vi "Read MasterConfiguration.vi"(7 "Action (Rd)":enum16{"Read", "Write"}(ring)=enum."Write", 8 "error in (no error)":errorcluster, 10 "MasterConfiguration":T1={"E109Configuration"={"PodPorts"=[{"portID"=101, "LocationID"="PodIn", "locationIndex"=1}, {"portID"=102, "LocationID"="PodOut", "locationIndex"=2}], "PodLocations"=["Buffer1", "Buffer2", "Buffer3", "Buffer4", "Buffer5", "Buffer6", "Buffer7", "Buffer8", "Buffer9", "Buffer10", "Buffer11", "Buffer12", "Buffer13", "Buffer14", "Buffer15", "Buffer16", "ASML1", "ASML2", "Manual"], "ReticleLocations"=[], "Opener1LocationID"="", "Opener2LocationID"="", "PodGantryArmLocationID"="", "VariableListPath"="", "EPJFilepath"=""}, "InBound"={"Simulation"=FALSE, "E84 Port Setup"={"Port ID"="", "baud rate"=9600, "data bits"=8, "parity"=enum."None", "stop bits"=10, "flow control"=0}, "UseVISAEvents"=FALSE, "Name"=""}, "OutBound"={"Simulation"=FALSE, "E84 Port Setup"={"Port ID"="", "baud rate"=9600, "data bits"=8, "parity"=enum."None", "stop bits"=10, "flow control"=0}, "UseVISAEvents"=FALSE, "Name"=""}, "InboundPodID"={"Simulation"=FALSE, "LoadPortCOM"={"VISA"="", "baud rate"=0, "data bits"=0, "parity"=enum."None", "flow control"=enum."None"}, "RFIDCOM"={"VISA"="", "baud rate"=0, "data bits"=0, "parity"=enum."None", "flow control"=enum."None"}, "SimulationRFID"=FALSE}, "OutboundPodID"={"Simulation"=FALSE, "LoadPortCOM"={"VISA"="", "baud rate"=0, "data bits"=0, "parity"=enum."None", "flow control"=enum."None"}, "RFIDCOM"={"VISA"="", "baud rate"=0, "data bits"=0, "parity"=enum."None", "flow control"=enum."None"}, "SimulationRFID"=FALSE}, "PBInterface"={"Simulation"=FALSE, "IPAddress"="", "StatusTag"="", "APIMoveTag"=""}} {"OutBound"."E84 Port Setup"."baud rate" items=["75"=75, "110"=110, "134"=134, "150"=150, "300"=300, "600"=600, "1200"=1200, "1800"=1800, "2400"=2400, "4800"=4800, "7200"=7200, "9600"=9600, "14400"=14400, "19200"=19200, "28800"=28800, "38400"=38400, "56000"=56000, "57600"=57600, "115200"=115200, "128000"=128000, "230400"=230400]; "OutBound"."E84 Port Setup"."flow control" items=["None", "XON/XOFF", "RTS/CTS", "XON/XOFF & RTS/CTS", "DTR/DSR", "XON/XOFF & DTR/DSR"]; "OutBound"."E84 Port Setup"."stop bits" items=["1"=10, "1.5"=15, "2"=20]; "OutBound"."E84 Port Setup"."data bits" min=5 max=8 step=1; "InBound"."E84 Port Setup"."baud rate" items=["75"=75, "110"=110, "134"=134, "150"=150, "300"=300, "600"=600, "1200"=1200, "1800"=1800, "2400"=2400, "4800"=4800, "7200"=7200, "9600"=9600, "14400"=14400, "19200"=19200, "28800"=28800, "38400"=38400, "56000"=56000, "57600"=57600, "115200"=115200, "128000"=128000, "230400"=230400]; "InBound"."E84 Port Setup"."flow control" items=["None", "XON/XOFF", "RTS/CTS", "XON/XOFF & RTS/CTS", "DTR/DSR", "XON/XOFF & DTR/DSR"]; "InBound"."E84 Port Setup"."stop bits" items=["1"=10, "1.5"=15, "2"=20]; "InBound"."E84 Port Setup"."data bits" min=5 max=8 step=1}, 11 "ConfigFile":path) -> (0 "error out":errorcluster, 2 "MasterConfigOut":T1={"E109Configuration"={"PodPorts"=[{"portID"=101, "LocationID"="PodIn", "locationIndex"=1}, {"portID"=102, "LocationID"="PodOut", "locationIndex"=2}], "PodLocations"=["Buffer1", "Buffer2", "Buffer3", "Buffer4", "Buffer5", "Buffer6", "Buffer7", "Buffer8", "Buffer9", "Buffer10", "Buffer11", "Buffer12", "Buffer13", "Buffer14", "Buffer15", "Buffer16", "ASML1", "ASML2", "Manual"], "ReticleLocations"=[], "Opener1LocationID"="", "Opener2LocationID"="", "PodGantryArmLocationID"="", "VariableListPath"="", "EPJFilepath"=""}, "InBound"={"Simulation"=FALSE, "E84 Port Setup"={"Port ID"="", "baud rate"=9600, "data bits"=8, "parity"=enum."None", "stop bits"=10, "flow control"=0}, "UseVISAEvents"=FALSE, "Name"=""}, "OutBound"={"Simulation"=FALSE, "E84 Port Setup"={"Port ID"="", "baud rate"=9600, "data bits"=8, "parity"=enum."None", "stop bits"=10, "flow control"=0}, "UseVISAEvents"=FALSE, "Name"=""}, "InboundPodID"={"Simulation"=FALSE, "LoadPortCOM"={"VISA"="", "baud rate"=0, "data bits"=0, "parity"=enum."None", "flow control"=enum."None"}, "RFIDCOM"={"VISA"="", "baud rate"=0, "data bits"=0, "parity"=enum."None", "flow control"=enum."None"}, "SimulationRFID"=FALSE}, "OutboundPodID"={"Simulation"=FALSE, "LoadPortCOM"={"VISA"="", "baud rate"=0, "data bits"=0, "parity"=enum."None", "flow control"=enum."None"}, "RFIDCOM"={"VISA"="", "baud rate"=0, "data bits"=0, "parity"=enum."None", "flow control"=enum."None"}, "SimulationRFID"=FALSE}, "PBInterface"={"Simulation"=FALSE, "IPAddress"="", "StatusTag"="", "APIMoveTag"=""}} {"OutBound"."E84 Port Setup"."baud rate" items=["75"=75, "110"=110, "134"=134, "150"=150, "300"=300, "600"=600, "1200"=1200, "1800"=1800, "2400"=2400, "4800"=4800, "7200"=7200, "9600"=9600, "14400"=14400, "19200"=19200, "28800"=28800, "38400"=38400, "56000"=56000, "57600"=57600, "115200"=115200, "128000"=128000, "230400"=230400]; "OutBound"."E84 Port Setup"."flow control" items=["None", "XON/XOFF", "RTS/CTS", "XON/XOFF & RTS/CTS", "DTR/DSR", "XON/XOFF & DTR/DSR"]; "OutBound"."E84 Port Setup"."stop bits" items=["1"=10, "1.5"=15, "2"=20]; "OutBound"."E84 Port Setup"."data bits" min=5 max=8 step=1; "InBound"."E84 Port Setup"."baud rate" items=["75"=75, "110"=110, "134"=134, "150"=150, "300"=300, "600"=600, "1200"=1200, "1800"=1800, "2400"=2400, "4800"=4800, "7200"=7200, "9600"=9600, "14400"=14400, "19200"=19200, "28800"=28800, "38400"=38400, "56000"=56000, "57600"=57600, "115200"=115200, "128000"=128000, "230400"=230400]; "InBound"."E84 Port Setup"."flow control" items=["None", "XON/XOFF", "RTS/CTS", "XON/XOFF & RTS/CTS", "DTR/DSR", "XON/XOFF & DTR/DSR"]; "InBound"."E84 Port Setup"."stop bits" items=["1"=10, "1.5"=15, "2"=20]; "InBound"."E84 Port Setup"."data bits" min=5 max=8 step=1})   [LabVIEW 2020]
uses:
  Controls/TD MasterConfiguration--cluster.ctl
  Subsystems/Cimetrix-main/Classes/TopLevel/Typedefs/E109Configuration--Cluster.ctl
  Subsystems/Cimetrix-main/Classes/TopLevel/Typedefs/E109_API_CreatePodPort_Data--Cluster.ctl
  Subsystems/Cimetrix-main/Classes/TopLevel/Typedefs/ToolModuleConfig--Cluster.ctl
  Subsystems/E84LoadPort/DataTypes/Settings--cluster.ctl
  Seminet_Common/DataTypes/serial_port_setup.ctl
  Subsystems/LoadPort/DataTypes/Settings--cluster.ctl
  Controls/TD SerialPortConfig--Cluster.ctl
  Subsystems/PodBufferInterface/DataTypes/Settings--cluster.ctl
  Subsystems/E84LoadPort/E84LoadPort.lvclass
  Subsystems/LoadPort/LoadPort.lvclass
  Subsystems/PodBufferInterface/PodBufferInterface.lvclass
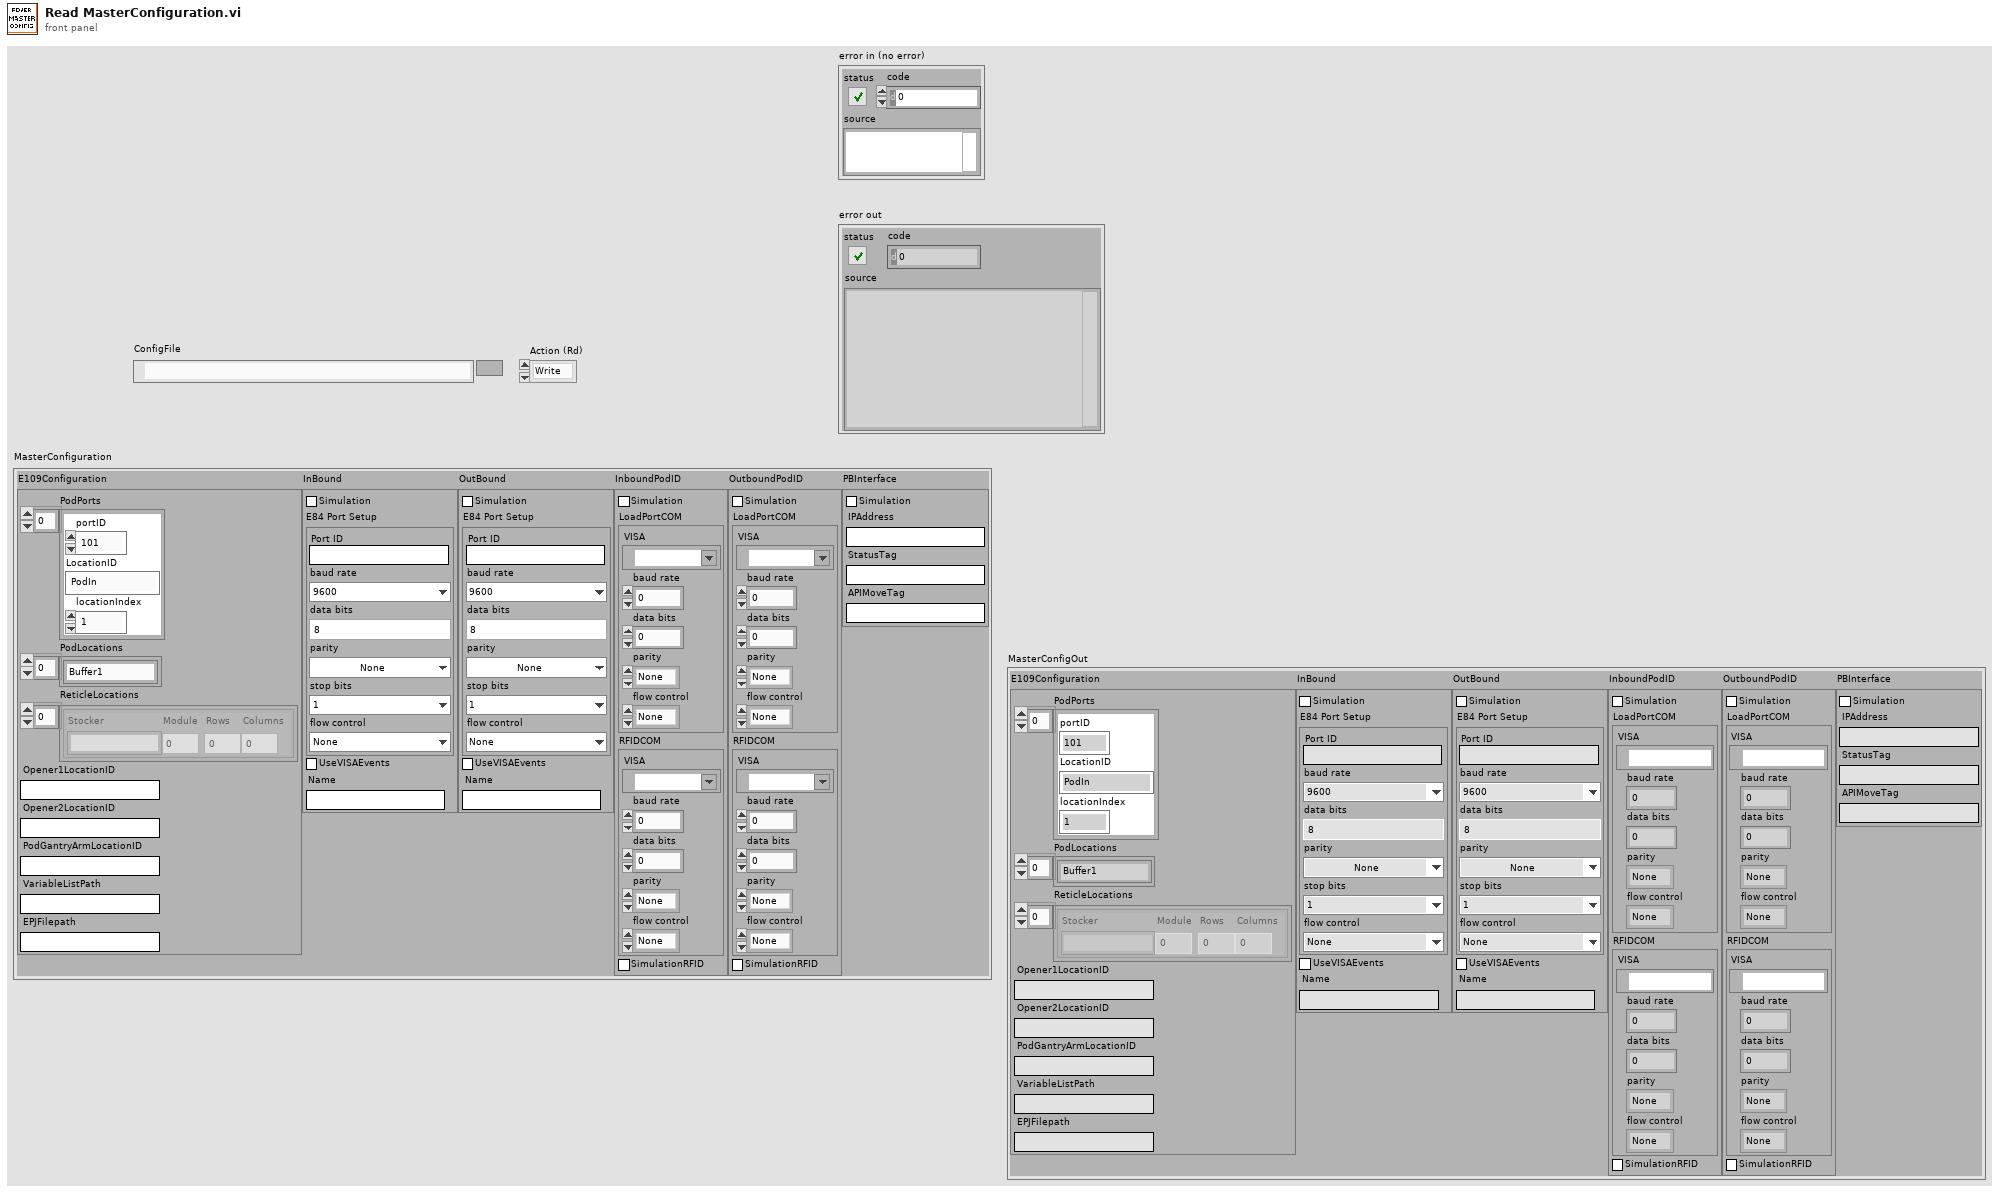
[diagram p1: front panel]
types:
  T1 = typedef "TD MasterConfiguration--cluster.ctl" = cluster{"E109Configuration":T2, "InBound":T5, "OutBound":T5, "InboundPodID":T7, "OutboundPodID":T7, "PBInterface":T9}
  T2 = typedef "E109Configuration--Cluster.ctl" = cluster{"PodPorts":T3[], "PodLocations":string[], "ReticleLocations":T4[], "Opener1LocationID":string, "Opener2LocationID":string, "PodGantryArmLocationID":string, "VariableListPath":string, "EPJFilepath":string}
  T3 = typedef "E109_API_CreatePodPort_Data--Cluster.ctl" = cluster{"portID":u8, "LocationID":string, "locationIndex":i32}
  T4 = typedef "ToolModuleConfig--Cluster.ctl" = cluster{"Stocker":string, "Module":u8, "Rows":u8, "Columns":u8}
  T5 = typedef "E84LoadPort.lvclass/Settings--cluster.ctl" = cluster{"Simulation":bool, "E84 Port Setup":T6, "UseVISAEvents":bool, "Name":string}
  T6 = typedef "serial_port_setup.ctl" = cluster{"Port ID":string, "baud rate":u32, "data bits":u16, "parity":enum16{"None", "Odd", "Even", "Mark", "Space"}, "stop bits":u16, "flow control":u16}
  T7 = typedef "LoadPort.lvclass/Settings--cluster.ctl" = cluster{"Simulation":bool, "LoadPortCOM":T8, "RFIDCOM":T8, "SimulationRFID":bool}
  T8 = typedef "TD SerialPortConfig--Cluster.ctl" = cluster{"VISA":refnum<visa-resource-name>, "baud rate":u32, "data bits":u16, "parity":enum16{"None", "Odd", "Even", "Mark", "Space"}, "flow control":enum16{"None", "XON/XOFF", "RTS/CTS", "XON/XOFF & RTS/CTS", "DTR/DSR", "XON/XOFF & DTR/DSR"}}
  T9 = typedef "PodBufferInterface.lvclass/Settings--cluster.ctl" = cluster{"Simulation":bool, "IPAddress":string, "StatusTag":string, "APIMoveTag":string}
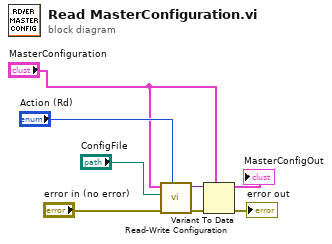
[diagram p0: block diagram]
diagram:
  n1 = call <vilib>:"Read-Write Configuration.vi"("TypedData in"="MasterConfiguration", "ConfigFile"="ConfigFile", "error in (no error)"="error in (no error)", "Action (Rd)"="Action (Rd)") -> ("Configuration Data out"=w6:variant, "error out"=w5:errorcluster)  [unwired: 2 in, 3 out]
  n2 = Variant To Data(error in=w5, type="MasterConfiguration", Variant=w6) -> (data=→"MasterConfigOut":T1, error out=→"error out":errorcluster)
